vi "GetXMLDeviceID.vi"(8 "error in":errorcluster, 11 "Node":refnum<k20>) -> (0 "error out":errorcluster, 3 "DeviceID":T1)   [LabVIEW 2013]
uses:
  <vilib>/xml/NI_XML.lvlib
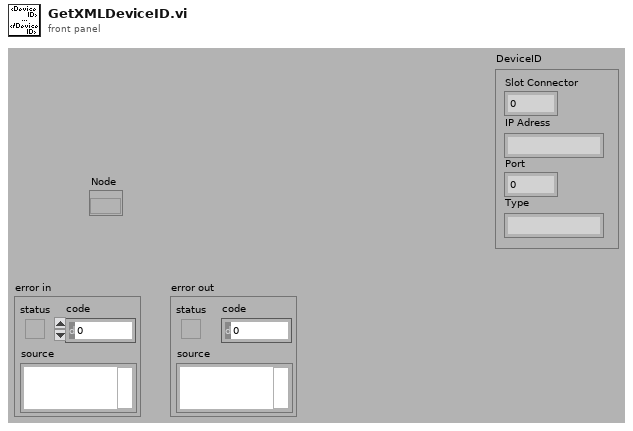
[diagram p1: front panel]
types:
  T1 = cluster{"Slot Connector":i32, "IP Adress":string, "Port":i32, "Type":string}
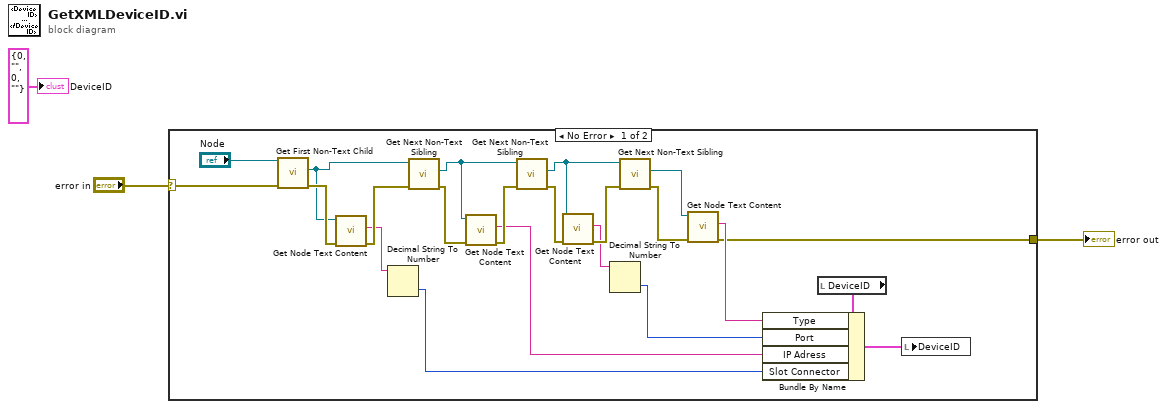
[diagram p0: block diagram]
diagram:
  n1 = case shown="No Error" "error in" {
    selector: "error in" -> [w5 w26]
    tunnel: [w6 w26] -> w2
    frame No Error {
      n2 = call <vilib>:"Get First Non-Text Child.vi"("error in (no error)"=w5, "node in"="Node") -> ("error out"=w24:errorcluster, "child node"=w4:refnum<k20>)  [unwired: 6 in, 2 out]
      n3 = call <vilib>:"Get Node Text Content.vi"("error in (no error)"=w24, "node in"=w4) -> ("error out"=w15:errorcluster, "node text"=w14:string)  [unwired: 7 in, 1 out]
      n4 = Decimal String To Number(string=w14) -> (number=w10:i32)  [unwired: 2 in, 1 out]
      n5 = call <vilib>:"Get Next Non-Text Sibling.vi"("error in (no error)"=w15, "node in"=w4) -> ("error out"=w23:errorcluster, "sibling node"=w18:refnum<k20>)  [unwired: 6 in, 2 out]
      n6 = call <vilib>:"Get Node Text Content.vi"("error in (no error)"=w23, "node in"=w18) -> ("error out"=w19:errorcluster, "node text"=w7:string)  [unwired: 7 in, 1 out]
      n7 = call <vilib>:"Get Next Non-Text Sibling.vi"("error in (no error)"=w19, "node in"=w18) -> ("error out"=w22:errorcluster, "sibling node"=w17:refnum<k20>)  [unwired: 6 in, 2 out]
      n8 = call <vilib>:"Get Node Text Content.vi"("error in (no error)"=w22, "node in"=w17) -> ("error out"=w20:errorcluster, "node text"=w13:string)  [unwired: 7 in, 1 out]
      n9 = Decimal String To Number(string=w13) -> (number=w8:i32)  [unwired: 2 in, 1 out]
      n10 = call <vilib>:"Get Next Non-Text Sibling.vi"("error in (no error)"=w20, "node in"=w17) -> ("error out"=w21:errorcluster, "sibling node"=w16:refnum<k20>)  [unwired: 6 in, 2 out]
      n11 = call <vilib>:"Get Node Text Content.vi"("error in (no error)"=w21, "node in"=w16) -> ("error out"=w6:errorcluster, "node text"=w9:string)  [unwired: 7 in, 1 out]
      n12 = local read "DeviceID"() -> (w12:T1)
      n13 = Bundle By Name(cluster=w12, "Type"=w9, "Port"=w8, "IP Adress"=w7, "Slot Connector"=w10) -> (w11:T1)
      n14 = local write "DeviceID"(w11) -> ()
    }
    frame Error {
    }
  }
  "error out" <- w2
  "DeviceID" <- T1 {"Slot Connector"=0, "IP Adress"="", "Port"=0, "Type"=""} ("DeviceID")
